vi "WSVCAP SHL Host TL RFFE Write - Single DUT.vi"(0 "Data Out":string, 11 "error in":errorcluster, 12 "Log (T)":bool=TRUE, 13 "DUT":T2, 14 "FPGA":T1) -> (15 "error out":errorcluster)   [LabVIEW 2012]
uses:
  Type Defs/WSVCAP SHL DUT Number Enum.ctl
  Type Defs/WSVCAP SHL I2C FPGA Enum.ctl
panel:
  out "Socket Mask":u64=1 format="%02x"
  out "RFFE Data Out":u8[][](array[numeric]) format="%02x"
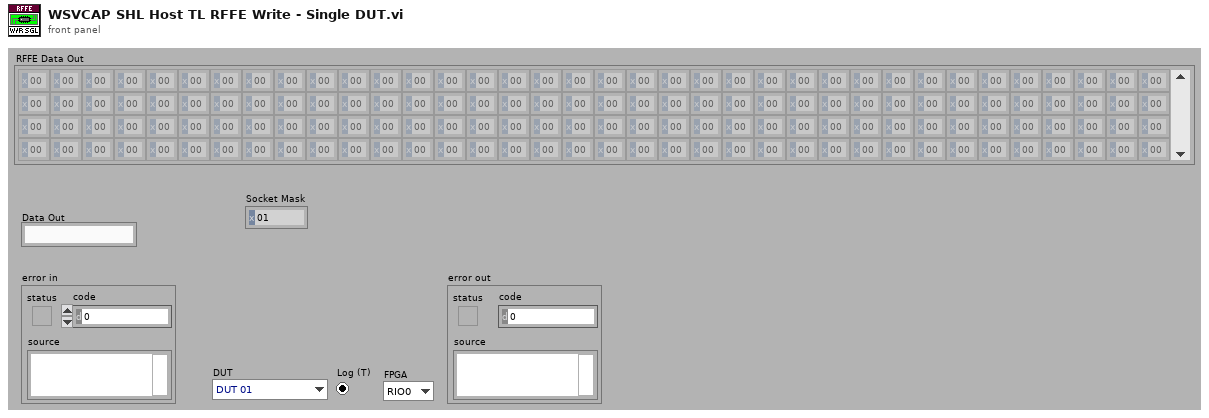
[diagram p1: front panel]
types:
  T1 = typedef "WSVCAP SHL I2C FPGA Enum.ctl" = enum16{"RIO0", "RIO1"}
  T2 = typedef "WSVCAP SHL DUT Number Enum.ctl" = enum16{"DUT 01", "DUT 02", "DUT 03", "DUT 04", "DUT 05", "DUT 06", "DUT 07", "DUT 08", "DUT 09", "DUT 10", "DUT 11", "DUT 12", "DUT 13", "DUT 14", "DUT 15", "DUT 16", "DUT 17", "DUT 18", "DUT 19", "DUT 20", "DUT 21", "DUT 22", "DUT 23", "DUT 24", "DUT 25", "DUT 26", "DUT 27", "DUT 28", "DUT 29", "DUT 30", "DUT 31", "DUT 32", "DUT 33", "DUT 34", "DUT 35", "DUT 36"}
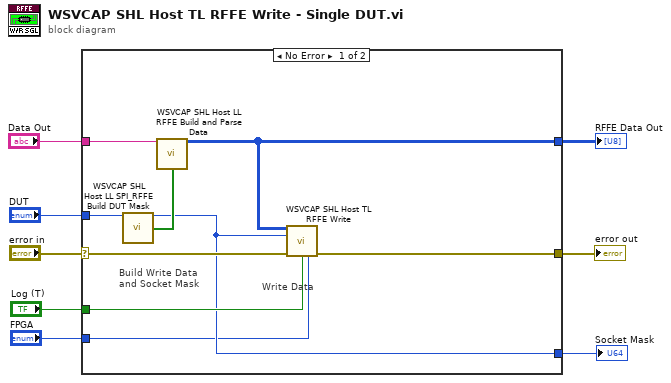
[diagram p0: block diagram]
diagram:
  n1 = case shown="No Error" "error in" {
    selector: "error in" -> [w16 _]
    tunnel: [w15 _] -> w8
    tunnel: "Data Out" -> [w14 _]
    tunnel: [w12 _] -> w5
    tunnel: "DUT" -> [w17 _]
    tunnel: [w10 _] -> w3
    tunnel: "Log (T)" -> [w11 _]
    tunnel: "FPGA" -> [w9 _]
    frame No Error {
      # "Write Data"
      # "Build Write Data and Socket Mask"
      n2 = call "WSVCAP SHL Host LL SPI_RFFE Build DUT Mask.vi"("DUT"=w17) -> ("Socket Mask [U64]"=w10:u64, "DUT Mask"=w13:bool[])  [unwired: 13 in]
      n3 = call "WSVCAP SHL Host LL RFFE Build and Parse Data.vi"("Data Out"=w14, "DUT Mask (All)"=w13) -> ("RFFE Data Out [U8]"=w12:u8[][])  [unwired: 10 in, 3 out]
      n4 = call "WSVCAP SHL Host TL RFFE Write.vi"("RFFE Data Out"=w12, "Socket Mask"=w10, "error in"=w16, "Log (T)"=w11, "FPGA"=w9) -> ("error out"=w15:errorcluster)  [unwired: 10 in]
    }
    frame Error {
    }
  }
  "error out" <- w8
  "RFFE Data Out" <- w5
  "Socket Mask" <- w3
